vi "Extract DOF Offset.vi"(1 "Combined":bool, 2 "IsForce":bool, 3 "LBCB Number":T1, 4 "Index":u32) -> (0 "DOF Value":dbl)   [LabVIEW 2009]
uses:
  Data Access Objects/Metadata/LBCB Number.ctl
  Global Data/Dataset Transaction Id.ctl
  Global Data/Dataset Source.ctl
  Global Data/Dataset Type.ctl
  Apps/Yes No Button.ctl
  Data Access Objects/Metadata/DAO Actions with Remove.ctl
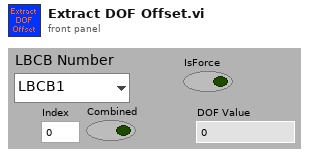
[diagram p1: front panel]
types:
  T1 = typedef "LBCB Number.ctl" = enum16{"LBCB1", "LBCB2"}
  T2 = typedef "DAO Actions with Remove.ctl" = enum16{"Init", "Get", "Set", "Remove"}
  T3 = typedef "Dataset Type.ctl" = enum16{"LVDT", "Load Cell", "Actuator Command", "Servo Error", "Displacement Command", "Displacement", "Force"}
  T4 = typedef "Dataset Transaction Id.ctl" = cluster{"Dataset Source":T5, "Dataset Type":T3, "Hold":T6, "Volts":T6, "Tag":string}
  T5 = typedef "Dataset Source.ctl" = enum16{"LBCB 1", "LBCB 2", "Combined", "External Sensors"}
  T6 = typedef "Yes No Button.ctl" = bool
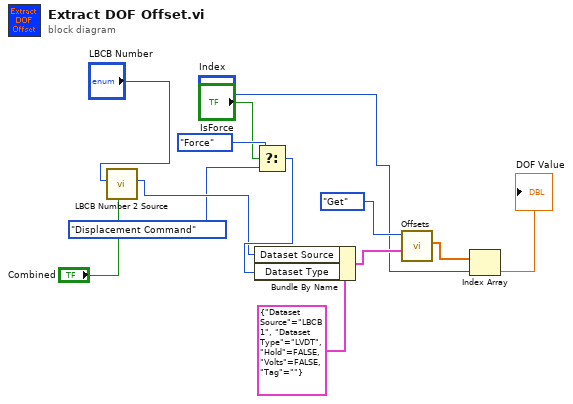
[diagram p0: block diagram]
diagram:
  n1 = call "LBCB Number 2 Source.vi"("Combined"="Combined", "LBCB Number"="LBCB Number") -> ("Dataset Source"=w9:T5)  [unwired: 9 in]
  n2 = Select(t=Dataset_Type."Force" ("Dataset Type"), s="IsForce", f=Dataset_Type."Displacement Command") -> (s? t:f=w10:T3)
  n3 = Bundle By Name(cluster=T4 {"Dataset Source"=enum."LBCB 1", "Dataset Type"=enum."LVDT", "Hold"=FALSE, "Volts"=FALSE, "Tag"=""} ("Dataset Trans Id"), "Dataset Source"=w9, "Dataset Type"=w10) -> (w12:T4)
  n4 = call "Offsets.vi"("Dataset Trans Id"=w12, "DAO Actions"=DAO_Actions_with_Remove."Get") -> ("Data Out"=w13:dbl[])  [unwired: 7 in, 2 out]
  n5 = Index Array(array=w13, index="Index") -> (element=→"DOF Value":dbl)
